vi "Cube Manipulation.vi"(8 "Spin Right":bool, 9 "Spin Left":bool, 10 "Outtake":bool, 11 "Intake":bool) -> ()   [LabVIEW 2017]
uses:
  <vilib>/Rock Robotics/WPI/ThirdParty/Phoenix-LabVIEW/Motor Controller/Controls/CTRE_Phoenix_MotorControl_ControlMode.ctl
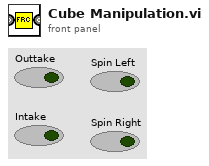
[diagram p1: front panel]
types:
  T1 = typedef "CTRE_Phoenix_MotorControl_ControlMode.ctl" = u16
  T2 = typedef "WPI_MotorControlDeviceRef.ctl" = cluster{"DeviceStatus":errorcluster, "Type":T3, "PWM":cluster{"PWM Channel":T4, "DeadBand":T5}, "CAN":cluster{"Device Number":u8, "SetOutput VI Ref":variant, "GetOutput VI Ref":variant, "Enable VI Ref":variant, "Disable VI Ref":variant, "Data":variant}, "Invert":bool, "DIO PWM":cluster{"PWM \"Enable\" Channel":T4, "DIOChannel":T6, "PWM Rate":dbl}}
  T3 = typedef "WPI_MotorControlType.ctl" = enum16{"PWM", "CAN", "DIO PWM"}
  T4 = typedef "FPGA_DIOPWMChannel.ctl" = enum8{"PWM 0", "PWM 1", "PWM 2", "PWM 3", "PWM 4", "PWM 5", "PWM 6", "PWM 7", "PWM 8", "PWM 9", "PWM MXP 0", "PWM MXP 1", "PWM MXP 2", "PWM MXP 3", "PWM MXP 4", "PWM MXP 5", "PWM MXP 6", "PWM MXP 7", "PWM MXP 8", "PWM MXP 9", "Invalid"}
  T5 = typedef "WPI_PWMDeadband.ctl" = cluster{"Name":string, "maxPositivePwm":i32, "minPositivePwm":i32, "centerPwm":i32, "maxNegativePwm":i32, "minNegativePwm":i32, "angularRange":u16}
  T6 = typedef "FPGA_DIOChannel.ctl" = enum8{"DIO 0", "DIO 1", "DIO 2", "DIO 3", "DIO 4", "DIO 5", "DIO 6", "DIO 7", "DIO 8", "DIO 9", "DIO MXP 0", "DIO MXP 1", "DIO MXP 2", "DIO MXP 3", "DIO MXP 4", "DIO MXP 5", "DIO MXP 6", "DIO MXP 7", "DIO MXP 8", "DIO MXP 9", "DIO MXP 10", "DIO MXP 11", "DIO MXP 12", "DIO MXP 13", "DIO MXP 14", "DIO MXP 15", "SPI Port CS1", "SPI Port CS2", "SPI Port CS3", "SPI Port MISO", "SPI Port MOSI", "Invalid"}
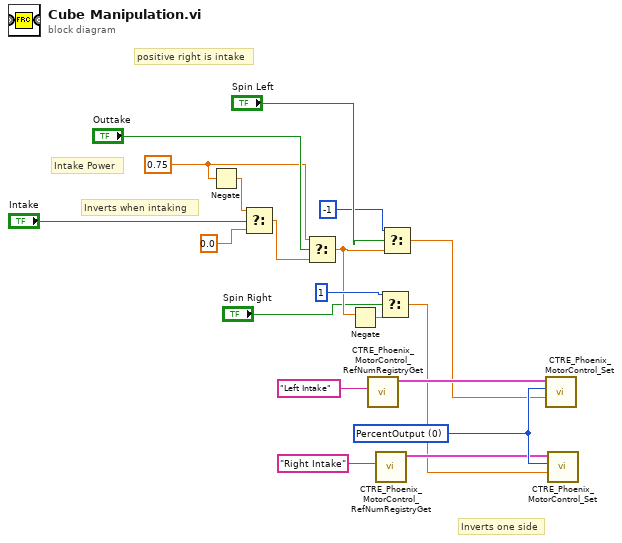
[diagram p0: block diagram]
diagram:
  w9 = 0.75 ("x")
  w16 = T1 0 items=["PercentOutput"=0, "Position"=1, "Velocity"=2, "Current"=3, "Follower"=5, "MotionProfile"=6, "MotionMagic"=7, "MotionMagicArc"=8, "MotionProfileArc"=10, "Disabled"=15] ("Control Mode")
  # "Inverts one side"
  # "Inverts when intaking"
  # "Intake Power"
  # "positive right is intake"
  n1 = Negate(x=w9) -> (-x=w19:dbl)
  n2 = Select(t=w19, s="Intake", f=0.0) -> (s? t:f=w18:dbl)
  n3 = Select(t=w9, s="Outtake", f=w18) -> (s? t:f=w3:dbl)
  n4 = Negate(x=w3) -> (-x=w2:dbl)
  n5 = call <vilib>:"CTRE_Phoenix_MotorControl_RefNumRegistryGet.vi"("refnum name"="Left Intake") -> ("PhoenixMotorControlDevRef"=w14:T2)  [unwired: 9 in, 1 out]
  n6 = call <vilib>:"CTRE_Phoenix_MotorControl_RefNumRegistryGet.vi"("refnum name"="Right Intake") -> ("PhoenixMotorControlDevRef"=w15:T2)  [unwired: 9 in, 1 out]
  n7 = Select(t=1, s="Spin Right", f=w2) -> (s? t:f=w7:dbl)
  n8 = Select(t=-1, s="Spin Left", f=w3) -> (s? t:f=w8:dbl)
  n9 = call <vilib>:"CTRE_Phoenix_MotorControl_Set.vi"("Output"=w8, "Control Mode"=w16, "PhoenixMotorControlDevRef"=w14) -> ()  [unwired: 7 in, 2 out]
  n10 = call <vilib>:"CTRE_Phoenix_MotorControl_Set.vi"("Output"=w7, "Control Mode"=w16, "PhoenixMotorControlDevRef"=w15) -> ()  [unwired: 7 in, 2 out]
